vi "Get Substep Index.vi"(8 "error in (no error)":errorcluster, 10 "Substep Name":string, 11 "Step in":refnum<class "Step.lvclass">) -> (0 "error out":errorcluster, 1 "Has Named Substep?":bool, 2 "Index":i32, 3 "Step out":refnum<class "Step.lvclass">)   [LabVIEW 2020, in "TSnax.lvlib" / "Step.lvclass"]
uses:
  Step.lvclass
  Step.lvclass/Step.ctl
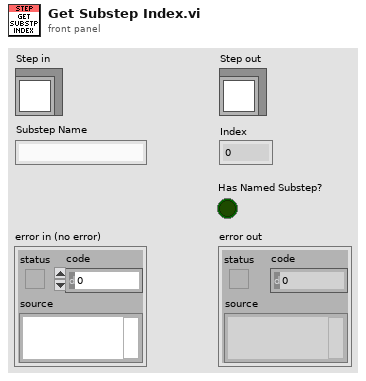
[diagram p1: front panel]
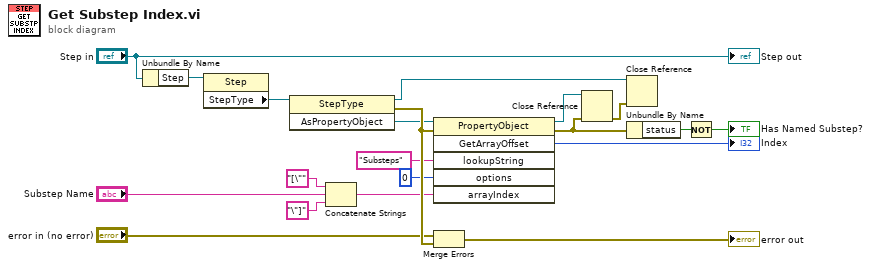
[diagram p0: block diagram]
diagram:
  n1 = Unbundle By Name("Step in") -> ("Step"=w16:refnum<k7>)
  n2 = property class="Step"(reference=w16) -> ("StepType"=w15:refnum<k7>)  [unwired: 1 in, 2 out]
  n3 = invoke class="StepType" method="AsPropertyObject"(reference=w15) -> (reference out=w3:refnum<k7>, error out=w20:errorcluster, "AsPropertyObject"=w12:refnum<k7>)  [unwired: 2 in]
  n4 = Concatenate Strings("[\"" ("string"), "Substep Name", "\"]" ("string")) -> (w7:string)
  n5 = invoke class="PropertyObject" method="GetArrayOffset"(reference=w12, error in=w20, "lookupString"="Substeps", "options"=0, "arrayIndex"=w7) -> (reference out=w14:refnum<k7>, error out=w6:errorcluster, "GetArrayOffset"=→"Index":i32)  [unwired: 1 in, 3 out]
  n6 = Merge Errors("error in (no error)", w20) -> (→"error out":errorcluster)
  n7 = Close Reference(reference=w14, error in (no error)=w6) -> (error out=w13:errorcluster)
  n8 = Close Reference(reference=w3, error in (no error)=w13) -> ()  [unwired: 1 out]
  n9 = Unbundle By Name(w6) -> ("status"=w5:bool)
  n10 = Not(x=w5) -> (.not. x?=→"Has Named Substep?":bool)
  "Step out" <- "Step in"
